vi "Estop.vi"() -> (2 "Estop?":bool)   [LabVIEW 2013]
panel:
  # "this is output\nsent to Teleop,\ndefaults to F"
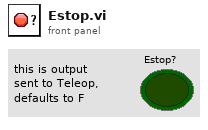
[diagram p1: front panel]
types:
  T1 = typedef "WPI_DigitalInputDevRef.ctl" = cluster{"DevStatus":errorcluster, "DIO Channel":T2, "Digital Module":T3}
  T2 = typedef "FPGA_DIOChannel.ctl" = enum8{"DIO 1", "DIO 2", "DIO 3", "DIO 4", "DIO 5", "DIO 6", "DIO 7", "DIO 8", "DIO 9", "DIO 10", "DIO 11", "DIO 12", "DIO 13", "DIO 14", "Invalid"}
  T3 = typedef "FPGA_TypedefDigitalModule.ctl" = enum16{"Digital Module 1", "Digital Module 2"}
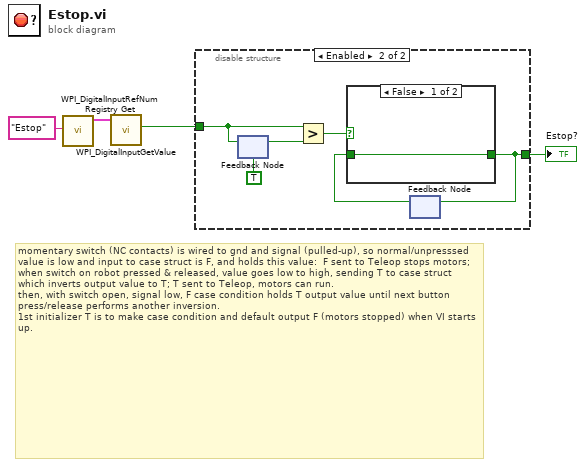
[diagram p0: block diagram]
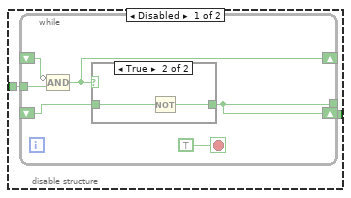
[diagram p2: hidden frame]
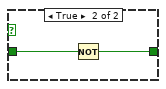
[diagram p4: hidden frame]
diagram:
  # "momentary switch (NC contacts) is wired to gnd and signal (pulled-up), so normal/unpresssed value is low and input to case struct is F, and holds this value:  F sent to Teleop stops motors;\nwhen switch on robot pressed & released, value goes low to high, sending T to case struct which inverts output value to T; T sent to Teleop, motors can run.\nthen, with switch open, signal low, F case condition holds T output value until next button press/release performs another inversion.\n1st initializer T is to make case condition and default output F (motors stopped) when VI starts up."
  n1 = call <vilib>:"WPI_DigitalInputRefNum Registry Get.vi"("refnum name"="Estop") -> ("DigitalInputDevRef"=w3:T1)  [unwired: 9 in, 1 out]
  n2 = call <vilib>:"WPI_DigitalInputGetValue.vi"("DigitalInputDevRef"=w3) -> ("Value"=w2:bool)  [unwired: 8 in, 2 out]
  n3 = disable-structure shown="Enabled" {
    disable-tunnel: w2 -> [w6 w20]
    disable-tunnel: [w5 w18] -> w1
    frame Disabled {
      n4 = while {
        tunnel: w6 -> [w12]
        tunnel: [w8] -> w5
        shift-right: [w8] -> _
        shift-left: _ -> [w9]
        shift-right: [w7] -> _
        shift-left: _ -> [w10]
        stop <- TRUE stop-if-true
        n5 = Compound Arithmetic op=AND(invert w10, w12) -> (w7:bool)
        n6 = case shown="True" w7 {
          tunnel: [w13 w15] -> w8
          tunnel: w9 -> [w13 w14]
          frame False {
          }
          frame True {
            n7 = Not(x=w14) -> (.not. x?=w15:bool)
          }
        }
      }
    }
    frame Enabled {
      n8 = feedback-in #1(w20) -> ()
      n9 = feedback #1(TRUE ("Value")) -> (w21:bool)
      n10 = Greater?(x=w20, y=w21) -> (0:w19:bool)
      n11 = feedback #2() -> (w17:bool)  [unwired: 1 in]
      n12 = case shown="False" w19 {
        tunnel: [w22 w23] -> w18
        tunnel: w17 -> [w22 w24]
        frame False {
        }
        frame True {
          n13 = Not(x=w24) -> (.not. x?=w23:bool)
        }
      }
      n14 = feedback-in #2(w18) -> ()
    }
  }
  "Estop?" <- w1
